vi "estimador de posicao.vi"(9 "life time":dbl, 10 "camera_id":u32, 11 "Detection Frame In":T1) -> (3 "estimador de frame":T1)   [LabVIEW 2016]
uses:
  SSL Detection Frame.ctl
  SSL Detection Robot.ctl
  SSL Detection Ball.ctl
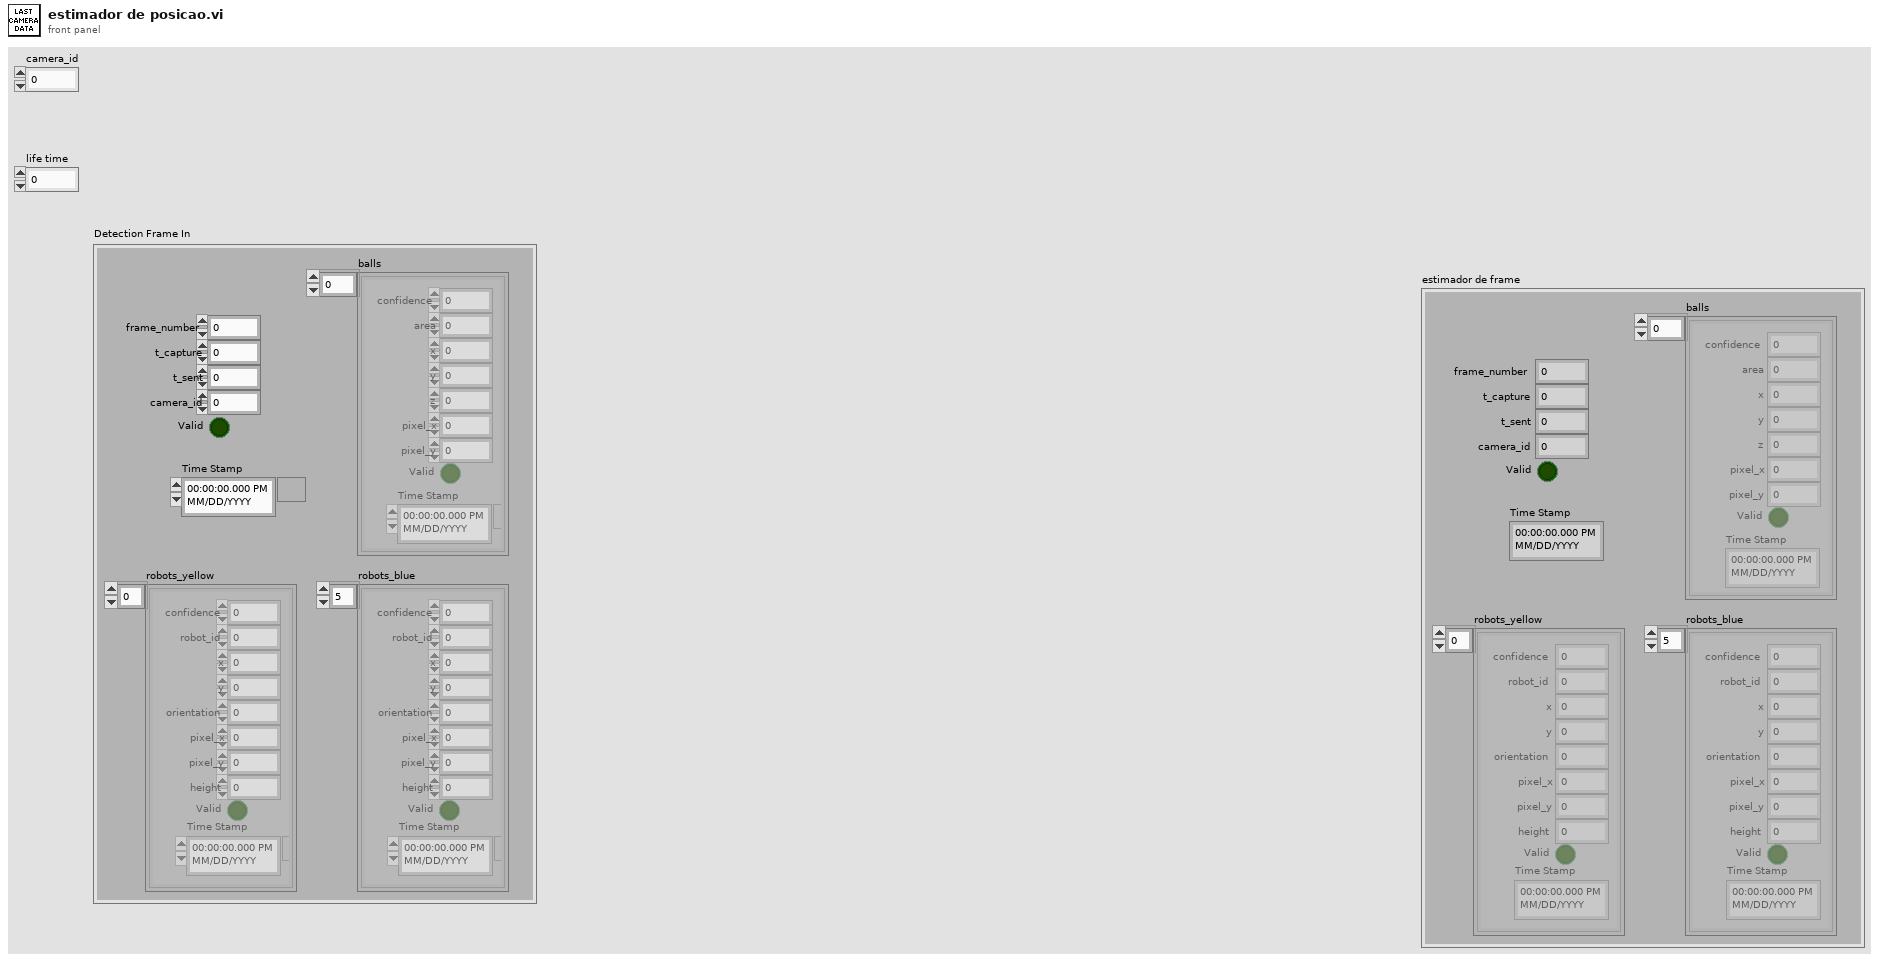
[diagram p1: front panel]
types:
  T1 = typedef "SSL Detection Frame.ctl" = cluster{"frame_number":u32, "t_capture":dbl, "t_sent":dbl, "camera_id":u32, "robots_yellow":T2[], "robots_blue":T2[], "balls":T3[], "Valid":bool, "Time Stamp":timestamp}
  T2 = typedef "SSL Detection Robot.ctl" = cluster{"x":dbl, "robot_id":u32, "confidence":sgl, "y":sgl, "orientation":sgl, "pixel_x":sgl, "pixel_y":sgl, "height":sgl, "Valid":bool, "Time Stamp":timestamp}
  T3 = typedef "SSL Detection Ball.ctl" = cluster{"x":sgl, "area":u32, "confidence":sgl, "y":sgl, "z":sgl, "pixel_x":sgl, "pixel_y":sgl, "Valid":bool, "Time Stamp":timestamp}
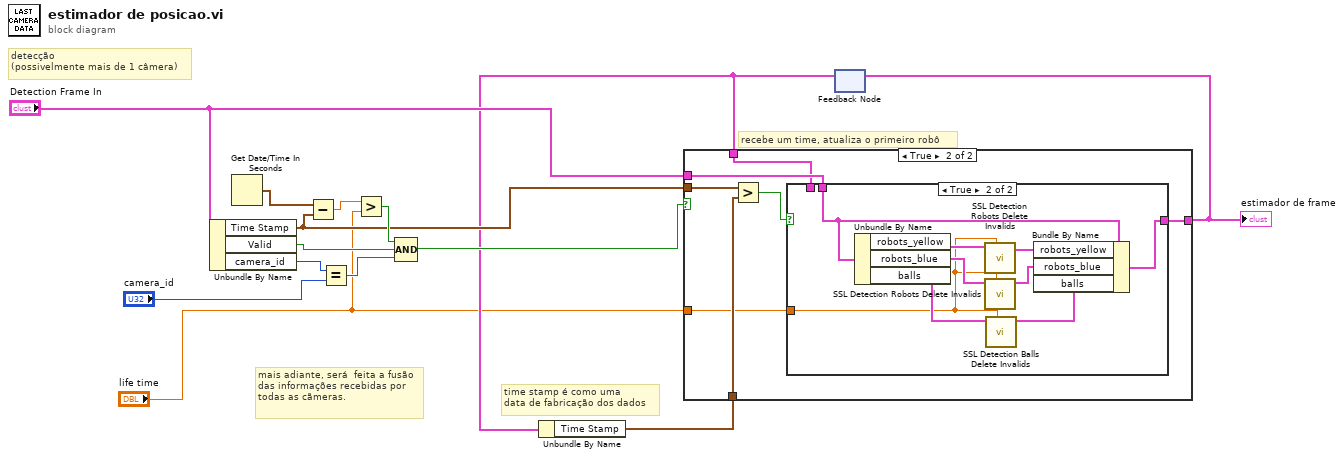
[diagram p0: block diagram]
diagram:
  # "recebe um time, atualiza o primeiro robô"
  # "time stamp é como uma\ndata de fabricação dos dados"
  # "mais adiante, será  feita a fusão das informações recebidas por todas as cãmeras."
  # "detecção\n(possivelmente mais de 1 câmera)"
  n1 = Unbundle By Name("Detection Frame In") -> ("Time Stamp"=w8:timestamp, "Valid"=w11:bool, "camera_id"=w13:u32)
  n2 = Get Date/Time In Seconds() -> (seconds since 1Jan1904=w5:timestamp)
  n3 = Subtract(x=w5, y=w8) -> (x-y=w10:dbl)
  n4 = Equal?(x=w13, y="camera_id") -> (x = y?=w12:bool)
  n5 = Greater?(x=w10, y="life time") -> (0:w9:bool)
  n6 = Compound Arithmetic op=AND(w9, w11, w12) -> (w7:bool)
  n7 = feedback #1() -> (w2:T1)  [unwired: 1 in]
  n8 = Unbundle By Name(w2) -> ("Time Stamp"=w6:timestamp)
  n9 = case shown="True" w7 {
    tunnel: w8 -> [_ w22]
    tunnel: w6 -> [_ w21]
    tunnel: [w15 w19] -> w3
    tunnel: "Detection Frame In" -> [_ w18]
    tunnel: w2 -> [w15 w17]
    tunnel: "life time" -> [_ w16]
    frame False {
    }
    frame True {
      n10 = Greater?(x=w22, y=w21) -> (0:w20:bool)
      n11 = case shown="True" w20 {
        tunnel: [w23 w25] -> w19
        tunnel: w18 -> [_ w29]
        tunnel: w17 -> [w23 _]
        tunnel: w16 -> [_ w24]
        frame False {
        }
        frame True {
          n12 = Unbundle By Name(w29) -> ("robots_yellow"=w32:T2[], "robots_blue"=w31:T2[], "balls"=w30:T3[])
          n13 = call "SSL Detection Robots Delete Invalids.vi"("Life Time"=w24, "Robots In"=w32) -> ("Robots Out"=w28:T2[])  [unwired: 9 in]
          n14 = call "SSL Detection Robots Delete Invalids.vi"("Life Time"=w24, "Robots In"=w31) -> ("Robots Out"=w27:T2[])  [unwired: 9 in]
          n15 = call "SSL Detection Balls Delete Invalids.vi"("Life Time"=w24, "Balls In"=w30) -> ("Balls Out"=w26:T3[])  [unwired: 9 in]
          n16 = Bundle By Name(cluster=w29, "robots_yellow"=w28, "robots_blue"=w27, "balls"=w26) -> (w25:T1)
        }
      }
    }
  }
  "estimador de frame" <- w3
  n17 = feedback-in #1(w3) -> ()
